vi "Register for Folder Path.vi"(8 "error in (no error)":errorcluster, 11 "Process Explorer View in":refnum<class "Process Explorer View.lvclass">) -> (0 "error out":errorcluster, 3 "Process Explorer View out":refnum<class "Process Explorer View.lvclass">)   [LabVIEW 2019, in "Process Explorer View.lvclass"]
doc: "<RequiredOverrideReason>Use this VI to register for Path to top level folder, or to hardcode the top level folder, whatever you want\nIf you use it to register then be sure to handle the registration in your code</RequiredOverrideReason>"
uses:
  <vilib>/gpm_packages/@cs/Car-wash/Source/Process Explorer View/Process Explorer View.lvclass
  C:/Program Files/National Instruments/LabVIEW 2019/vi.lib/gpm_packages/@cs/file-explorer-extension/Source/File Explorer/File Explorer/File Explorer.lvclass
  <vilib>/gpm_packages/@cs/file-explorer-extension/Source/File Explorer/File Explorer/File Explorer.lvclass
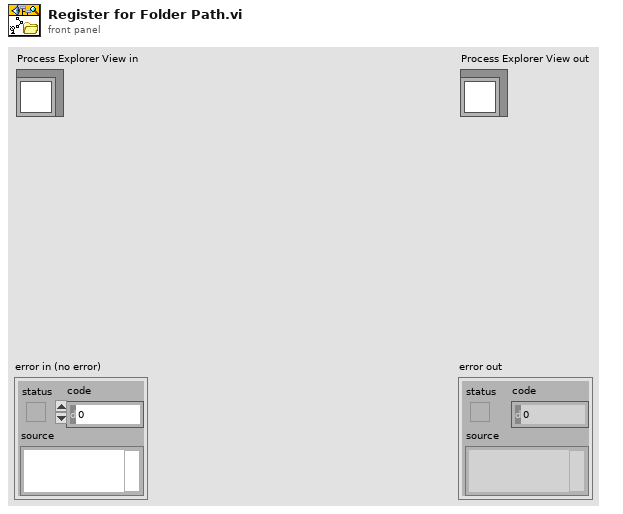
[diagram p1: front panel]
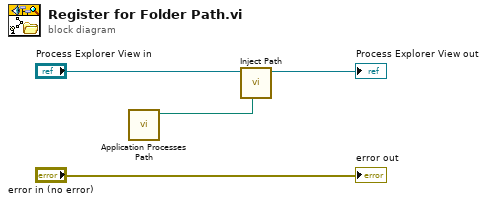
[diagram p0: block diagram]
diagram:
  n1 = call <vilib>:"Application Processes Path.vi"() -> ("Application Processes Path"=w2:path)  [unwired: 11 in]
  n2 = call <vilib>:"Inject Path.vi"("Path"=w2, "File Explorer in"="Process Explorer View in") -> ("File Explorer out"=→"Process Explorer View out":refnum<class "Process Explorer View.lvclass">)  [unwired: 9 in]
  "error out" <- "error in (no error)"
